vi "Test_tcp_client.vi"(6 "close_tcp":bool=TRUE, 7 "wait_time":i32=1000, 8 "error in":errorcluster, 9 "port":u16=9999, 10 "address":string="127.0.0.1", 11 "conn_id_in":refnum<k5>) -> (0 "error out":errorcluster, 1 "array_value":dbl[](array[numeric]), 2 "data":string, 3 "conn_id_out":refnum<k5>, 4 "status":bool)   [LabVIEW 2019]
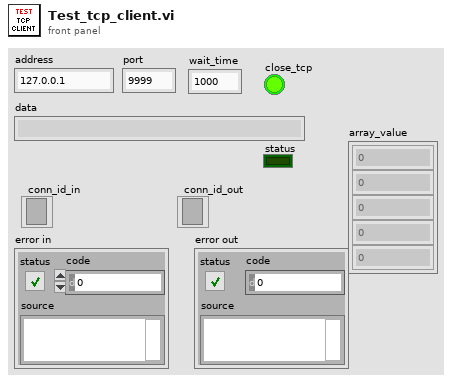
[diagram p1: front panel]
types:
  T1 = enum16{"Standard", "Buffered", "CRLF", "Immediate"}
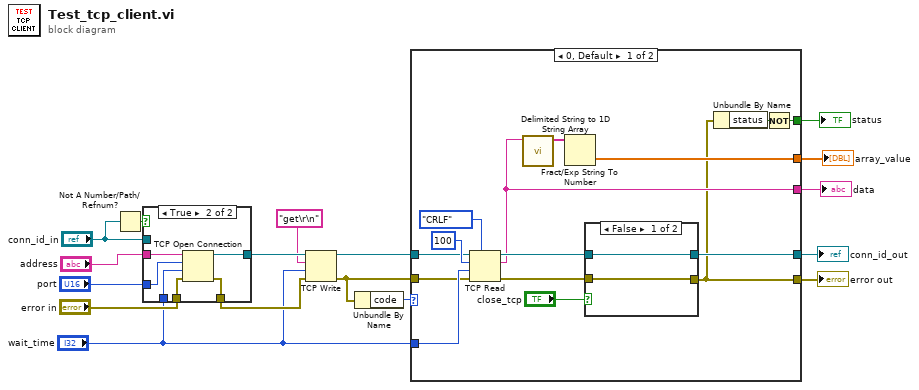
[diagram p0: block diagram]
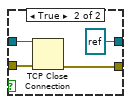
[diagram p2: hidden frame]
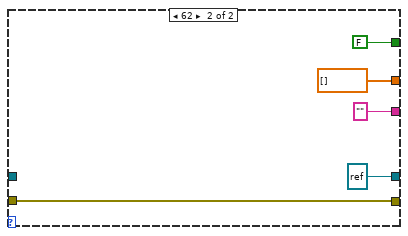
[diagram p3: hidden frame]
diagram:
  n1 = Not A Number/Path/Refnum?(number/path/refnum="conn_id_in") -> (NaN/Path/Refnum?=w16:bool)
  n2 = case shown="True" w16 {
    tunnel: "port" -> [_ w21]
    tunnel: "address" -> [_ w25]
    tunnel: [w18 w24] -> w9
    tunnel: [w19 w23] -> w11
    tunnel: "conn_id_in" -> [w19 _]
    tunnel: "error in" -> [w18 w22]
    tunnel: "wait_time" -> [_ w20]
    frame False {
    }
    frame True {
      n3 = TCP Open Connection(address=w25, remote port or service name=w21, timeout ms (60000)=w20, error in (no error)=w22) -> (connection ID=w23:refnum<k5>, error out=w24:errorcluster)  [unwired: 1 in]
    }
  }
  n4 = TCP Write(connection ID=w11, data in="get\r\n", error in (no error)=w9, 9:"wait_time") -> (connection ID out=w7:refnum<k5>, error out=w4:errorcluster)  [unwired: 1 out]
  n5 = Unbundle By Name(w4) -> ("code"=w3:i32)
  n6 = case shown="0, Default" w3 {
    tunnel: [w27 FALSE] -> w17
    tunnel: "wait_time" -> [w36 _]
    tunnel: w7 -> [w35 _]
    tunnel: [w33 refnum<k5> refnum ("connection ID")] -> w6
    tunnel: [w28 w51] -> w5
    tunnel: w4 -> [w32 w51]
    tunnel: [w31 dbl[] []] -> w2
    tunnel: [w29 "" ("data out")] -> w1
    frame 0, Default {
      n7 = TCP Read(connection ID=w35, bytes to read=100, error in (no error)=w32, 7:T1."CRLF" ("mode (standard)"), 9:w36) -> (connection ID out=w39:refnum<k5>, data out=w29:string, error out=w40:errorcluster)
      n8 = call <vilib>:"Delimited String to 1D String Array.vi"("delimited string"=w29) -> ("string array"=w30:string[])  [unwired: 10 in]
      n9 = Fract/Exp String To Number(string=w30) -> (number=w31:dbl[])  [unwired: 3 in, 1 out]
      n10 = case shown="False" "close_tcp" {
        tunnel: w40 -> [w41 w46]
        tunnel: w39 -> [w42 w45]
        tunnel: [w41 w44] -> w28
        tunnel: [w42 refnum<k5> refnum ("connection ID")] -> w33
        frame False {
        }
        frame True {
          n11 = TCP Close Connection(connection ID=w45, error in (no error)=w46) -> (error out=w44:errorcluster)  [unwired: 1 in, 1 out]
        }
      }
      n12 = Unbundle By Name(w28) -> ("status"=w26:bool)
      n13 = Not(x=w26) -> (.not. x?=w27:bool)
    }
    frame 62 {
    }
  }
  "status" <- w17
  "conn_id_out" <- w6
  "error out" <- w5
  "array_value" <- w2
  "data" <- w1
